vi "Send UI_ShowIn_Subpanel.vi"(7 "Message Priority (Normal)":T1=enum."Normal", 8 "error in (no error)":errorcluster, 10 "Sub Panel":refnum<vi>, 11 "Message Enqueuer":refnum<class "Message Enqueuer.lvclass">) -> (0 "error out":errorcluster, 3 "Message Enqueuer out":refnum<class "Message Enqueuer.lvclass">)   [LabVIEW 2020, in "UI_Actor.lvlib" / "UI_ShowIn_Subpanel Msg.lvclass"]
doc: "This VI sends the message to an actor."
uses:
  UI_ShowIn_Subpanel Msg.lvclass
  support/Actor Framework.lvlibp/1abvi3w/vi.lib/ActorFramework/Message Enqueuer/Message Enqueuer.lvclass
  D:/Elie/Documents/ui-actor/support/Actor Framework.lvlibp/1abvi3w/vi.lib/ActorFramework/Message/Message.lvclass
  D:/Elie/Documents/ui-actor/UI_Actor/UI_Actor Messages/UI_ShowIn_Subpanel Msg/UI_ShowIn_Subpanel Msg.lvclass
  support/Actor Framework.lvlibp/1abvi3w/vi.lib/ActorFramework/Message Enqueuer/Message Priority.ctl
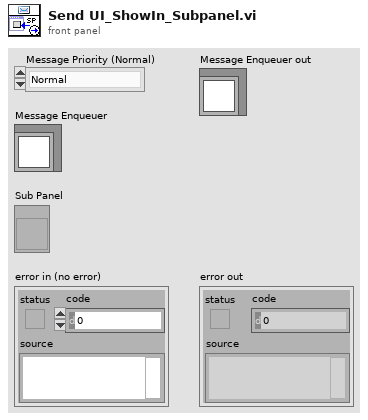
[diagram p1: front panel]
types:
  T1 = typedef "Actor Framework.lvlibp/Message Enqueuer.lvclass/Message Priority.ctl" = enum16{"Low", "Normal", "High"}
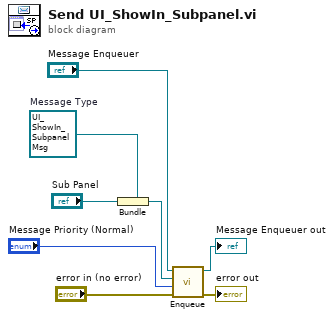
[diagram p0: block diagram]
diagram:
  w2 = refnum<class "UI_ShowIn_Subpanel Msg.lvclass"> refnum  # Message Type
  n1 = Bundle(cluster=w2, "Sub Panel") -> (w3:refnum<class "UI_ShowIn_Subpanel Msg.lvclass">)
  n2 = call "Enqueue.vi"("error in (no error)"="error in (no error)", "Message Priority (Normal)"="Message Priority (Normal)", "Message"=w3, "Message Enqueuer in"="Message Enqueuer") -> ("error out"=→"error out":errorcluster, "Message Enqueuer in"=→"Message Enqueuer out":refnum<class "Message Enqueuer.lvclass">)  [unwired: 6 in]
